vi "IMUcalc Bias.vi"(7 "Number of loops":i32, 10 "error in (no error)":errorcluster) -> (1 "Bias":T1, 3 "error out":errorcluster)   [LabVIEW 2016]
doc: "Inputs\nNumber of loops\n\nOutputs\nBias\n\nThis VI calculates the bias for the accelerometer and gyroscopic readings, the bias is later used when the lean angle is calculated. When this VI runs it is important that the bicycle stands still in an upright position so the IMU values are as accurate as possible."
panel:
  out "Z gyro bias":dbl
  out "Y gyro bias":dbl
  out "X gyro bias":dbl
  out "Z acc bias":dbl
  out "Y acc bias":dbl
  out "X acc bias":dbl
  out "Accel, Gyro":u16[](array[numeric])
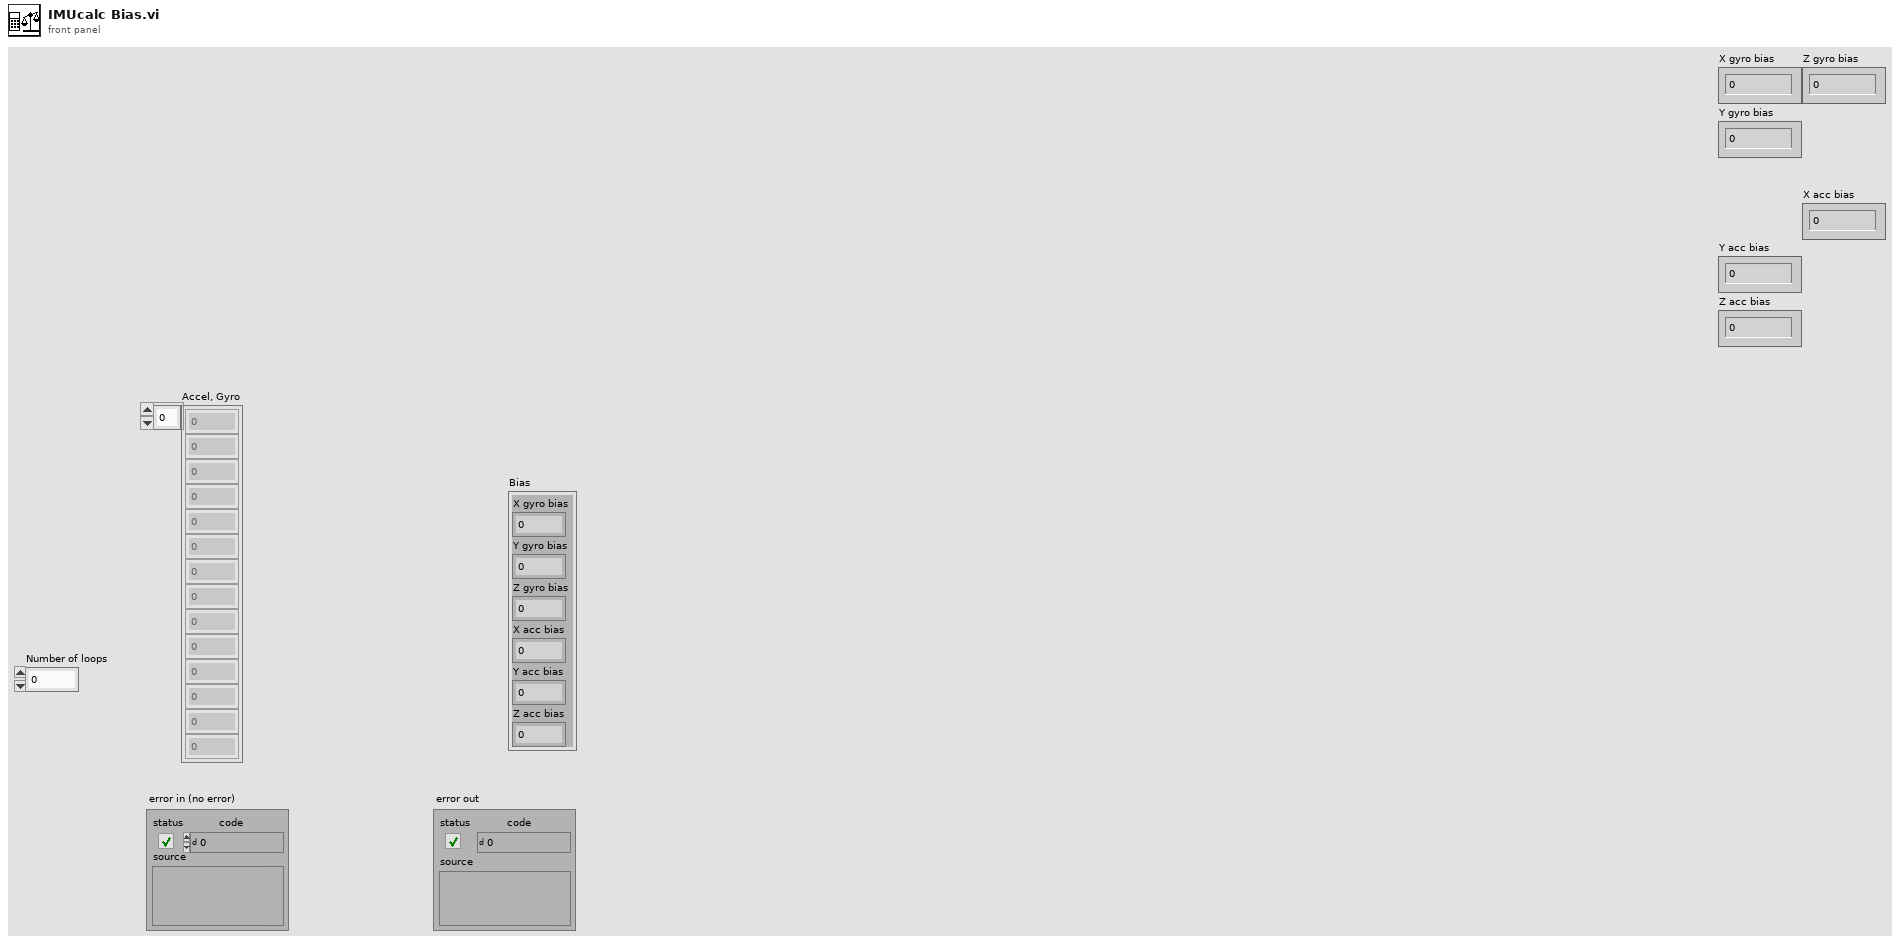
[diagram p1: front panel]
types:
  T1 = cluster{"X gyro bias":dbl, "Y gyro bias":dbl, "Z gyro bias":dbl, "X acc bias":dbl, "Y acc bias":dbl, "Z acc bias":dbl}
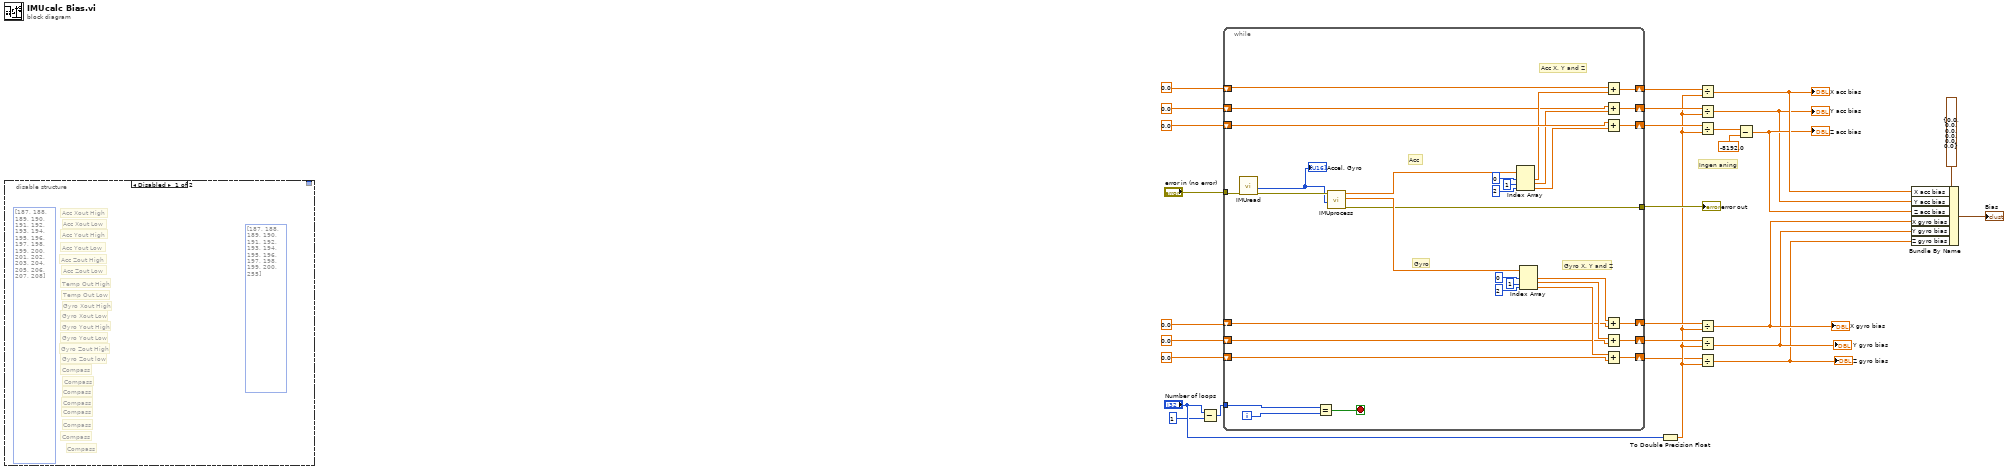
[diagram p0: block diagram]
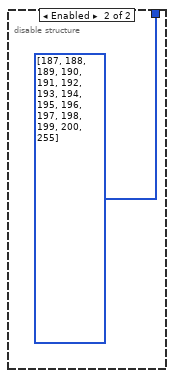
[diagram p2: hidden frame]
diagram:
  # "Ingen aning"
  n1 = disable-structure shown="Disabled" {
    disable-tunnel: [_ u16[] [187, 188, 189, 190, 191, 192, 193, 194, 195, 196, 197, 198, 199, 200, 255] ("Frames to Write")] -> _
    frame Disabled {
      (unwired) u16[] [187, 188, 189, 190, 191, 192, 193, 194, 195, 196, 197, 198, 199, 200, 201, 202, 203, 204, 205, 206, 207, 208] ("Frames to Write")
      (unwired) u16[] [187, 188, 189, 190, 191, 192, 193, 194, 195, 196, 197, 198, 199, 200, 255] ("Frames to Write")
      # "Compass"
      # "Compass"
      # "Compass"
      # "Compass"
      # "Compass"
      # "Compass"
      # "Compass"
      # "Compass"
      # "Gyro Zout low"
      # "Gyro Zout High"
      # "Gyro Yout Low"
      # "Gyro Yout High"
      # "Gyro Xout Low"
      # "Gyro Xout High"
      # "Temp Out Low"
      # "Temp Out High"
      # "Acc Zout Low"
      # "Acc Zout High"
      # "Acc Yout Low"
      # "Acc Yout High"
      # "Acc Xout Low"
      # "Acc Xout High"
    }
    frame Enabled {
    }
  }
  n2 = Subtract(x="Number of loops", y=1) -> (x-y=w2:i32)
  n3 = while {
    shift-right: [w52] -> w20
    shift-left: 0.0 -> [w54]
    shift-right: [w51] -> w19
    shift-left: 0.0 -> [w48]
    shift-right: [w50] -> w18
    shift-left: 0.0 -> [w53]
    tunnel: [w45] -> w25
    tunnel: "error in (no error)" -> [w44]
    shift-right: [w43] -> w17
    shift-left: 0.0 -> [w37]
    shift-right: [w42] -> w16
    shift-left: 0.0 -> [w36]
    shift-right: [w41] -> w4
    shift-left: 0.0 -> [w35]
    tunnel: w2 -> [w31]
    i -> [w34]
    stop <- w30 stop-if-true
    # "Gyro"
    # "Acc"
    # "Gyro X, Y and Z"
    # "Acc X, Y and Z"
    n4 = call "IMUread.vi"("error in (no error)"=w44) -> ("error out"=w62:errorcluster, "Accel, Gyro"=w33:u16[])  [unwired: 9 in]
    "Accel, Gyro" <- w33
    n5 = Equal?(x=w31, y=w34) -> (x = y?=w30:bool)
    n6 = call "IMUprocess.vi"("Frames Read"=w33, "error in (no error)"=w62) -> ("error out"=w45:errorcluster, "Gyro deg/s"=w59:dbl[], "Accel g's"=w32:dbl[])  [unwired: 7 in]
    n7 = Index Array(array=w32, index #1=0 ("index"), index #2=1 ("index"), index #3=2 ("index")) -> (element #1=w49:dbl, element #2=w47:dbl, element #3=w46:dbl)
    n8 = Index Array(array=w59, index #1=0 ("index"), index #2=1 ("index"), index #3=2 ("index")) -> (element #1=w40:dbl, element #2=w39:dbl, element #3=w38:dbl)
    n9 = Add(x=w54, y=w49) -> (x+y=w52:dbl)
    n10 = Add(x=w48, y=w47) -> (x+y=w51:dbl)
    n11 = Add(x=w53, y=w46) -> (x+y=w50:dbl)
    n12 = Add(x=w40, y=w37) -> (x+y=w43:dbl)
    n13 = Add(x=w39, y=w36) -> (x+y=w42:dbl)
    n14 = Add(x=w38, y=w35) -> (x+y=w41:dbl)
  }
  "error out" <- w25
  n15 = To Double Precision Float(number="Number of loops") -> (double precision float=w5:dbl)
  n16 = Divide(x=w20, y=w5) -> (x/y=w12:dbl)
  "X acc bias" <- w12
  n17 = Divide(x=w19, y=w5) -> (x/y=w7:dbl)
  "Y acc bias" <- w7
  n18 = Divide(x=w18, y=w5) -> (x/y=w10:dbl)
  n19 = Divide(x=w17, y=w5) -> (x/y=w15:dbl)
  "X gyro bias" <- w15
  n20 = Divide(x=w16, y=w5) -> (x/y=w14:dbl)
  "Y gyro bias" <- w14
  n21 = Divide(x=w4, y=w5) -> (x/y=w13:dbl)
  "Z gyro bias" <- w13
  n22 = Subtract(x=w10, y=-8192.0) -> (x-y=w9:dbl)
  "Z acc bias" <- w9
  n23 = Bundle By Name(cluster=T1 {"X gyro bias"=0.0, "Y gyro bias"=0.0, "Z gyro bias"=0.0, "X acc bias"=0.0, "Y acc bias"=0.0, "Z acc bias"=0.0} ("Cluster"), "X acc bias"=w12, "Y acc bias"=w7, "Z acc bias"=w9, "X gyro bias"=w15, "Y gyro bias"=w14, "Z gyro bias"=w13) -> (→"Bias":T1)
